vi "HAL Camera specifications globals - SubVI.vi"() -> ()   [LabVIEW 2014]
panel:
  in  "Camera Name":string="Andor iXon 512"
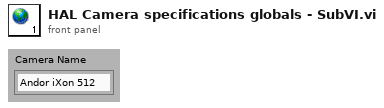
[diagram p1: front panel]
diagram:
